vi "Lookup Group.vi"(7 "Group Type (Abstract)":refnum<class "Group.lvclass">, 8 "error in (no error)":errorcluster, 10 "Group Name":string, 11 "VolatusAPI":refnum<class "VolatusAPI.lvclass">) -> (0 "error out":errorcluster, 2 "Group":refnum<class "Group.lvclass">)   [LabVIEW 2020, in "VolatusGUI.lvlib"]
uses:
  VolatusGUI.lvlib
  Volatus/VolatusAPI/VolatusAPI.lvclass
  VolatusConfig/Node/Node Config.lvclass
  VolatusConfig/Cluster/Cluster Config.lvclass
  lv-vecto/Vecto/Group/Group.lvclass
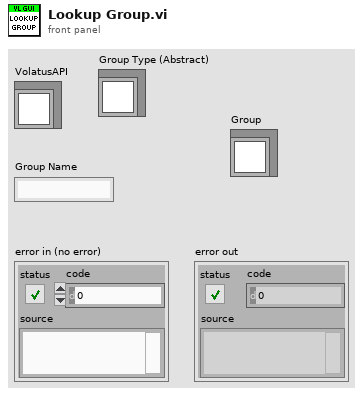
[diagram p1: front panel]
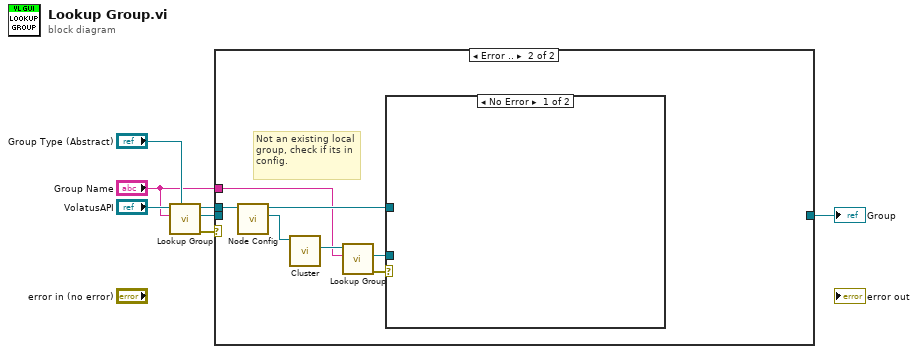
[diagram p0: block diagram]
diagram:
  n1 = call "Lookup Group.vi"("Group Type (Abstract)"="Group Type (Abstract)", "Group Name"="Group Name", "VolatusAPI in"="VolatusAPI") -> ("error out"=w5:errorcluster, "Group"=w3:refnum<class "Group.lvclass">, "VolatusAPI out"=w4:refnum<class "VolatusAPI.lvclass">)  [unwired: 6 in]
  n2 = case shown="Error .." w5 {
    tunnel: w4 -> [_ w15]
    tunnel: w3 -> [w8 _]
    tunnel: [w8 _] -> w2
    tunnel: "Group Name" -> [_ w11]
    frame No Error {
    }
    frame Error {
      # "Not an existing local group, check if its in config."
      n3 = call "Node Config.vi"("VolatusAPI in"=w15) -> ("Node Config"=w14:refnum<class "Node Config.lvclass">, "VolatusAPI out"=w13:refnum<class "VolatusAPI.lvclass">)  [unwired: 9 in]
      n4 = call "Cluster.vi"("Node in"=w14) -> ("Cluster"=w12:refnum<class "Cluster Config.lvclass">)  [unwired: 8 in, 2 out]
      n5 = call "Lookup Group.vi"("Group Name"=w11, "Cluster in"=w12) -> ("error out"=w10:errorcluster, "Group"=w9:refnum<class "Group Config.lvclass">)  [unwired: 6 in, 2 out]
      n6 = case shown="No Error" w10 {
        tunnel: w13 -> [_ _]
        tunnel: w9 -> [_ _]
        frame No Error {
        }
        frame Error {
        }
      }
    }
  }
  "Group" <- w2
